vi "Configure Cells.vi"(8 "error in":errorcluster, 10 "dt":dbl, 11 "cCRDS in":refnum<class "cCRDS.lvclass">=refnum) -> (0 "error out":errorcluster, 3 "cCRDS out":refnum<class "cCRDS.lvclass">)   [LabVIEW 2015, in "cCRDS.lvclass"]
uses:
  cCRDS.lvclass
  Reusable/CRDS/Cell/CRDS Cell.lvclass
  Reusable/CRDS/Data/Cell/CRDS Cell Data.lvclass
  Reusable/CRDS/Data/Main/CRDS Data.lvclass
  Reusable/CRDS/Cell/Get Tau Method.ctl
  Data/cCRDS Data.lvclass
  Reusable/CRDS/Cell/CRDS Cell.lvclass/CRDS Cell.ctl
  Reusable/CRDS/Cell/Read Data.vi
  Reusable/CRDS/Cell/Write aVar Params.vi
  Reusable/CRDS/Cell/Write Data.vi
  Reusable/General/Atmospheric/Atmospheric Constants.vi
  Reusable/CRDS/Cell/Write CalType.vi
  Reusable/CRDS/Cell/Write errorCalOn.vi
  Reusable/CRDS/Cell/Write optTimeConst.vi
  Reusable/CRDS/Cell/Write dt.vi
  Reusable/CRDS/Cell/Write lambda.vi
  Reusable/CRDS/Data/Main/Write CellData.vi
  Reusable/CRDS/Main/Write Data.vi
  Reusable/CRDS/Main/Write Cells.vi
  Reusable/General/Atmospheric/Atmospheric Library.lvlib
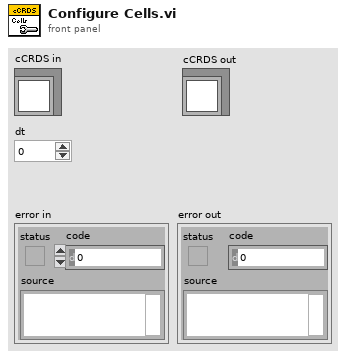
[diagram p1: front panel]
types:
  T1 = cluster{"tmeas":dbl, "tint":sgl[], "ttot":dbl, "Varaince On":bool}
  T2 = typedef "Get Tau Method.ctl" = enum8{"DFT-1", "DFT-5", "LRS"}
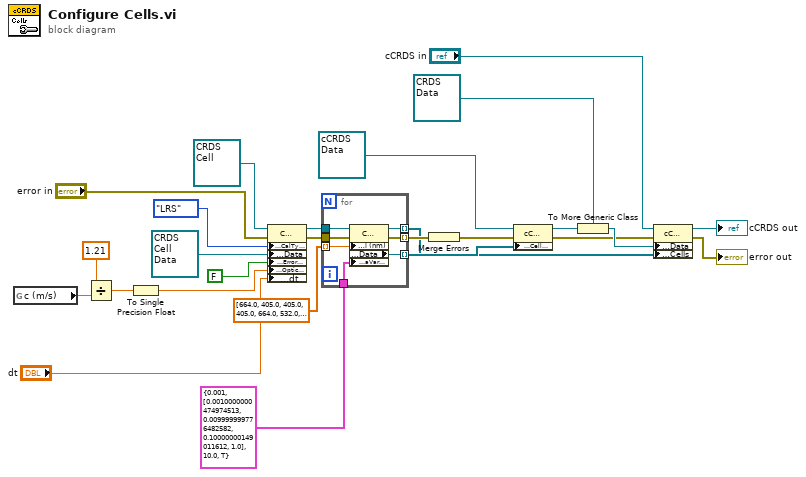
[diagram p0: block diagram]
diagram:
  n1 = global read "Atmospheric Constants.vi" "c (m/s)"() -> (w13:dbl)
  n2 = Divide(x=1.21, y=w13) -> (x/y=w14:dbl)
  n3 = To Single Precision Float(number=w14) -> (single precision float=w20:sgl)
  n4 = property class="CRDS Cell"(reference=refnum<class "CRDS Cell.lvclass"> refnum ("CRDS Cell"), error in="error in", "Data Access:CalType"=Get_Tau_Method."LRS" ("CalType"), "Data Access:Data"=refnum<class "CRDS Cell Data.lvclass"> refnum ("CRDS Cell"), "Data Access:Error Cal On?"=FALSE ("Error Cal On?"), "Data Access:Optical Time Constant"=w20, "Data Access:dt"="dt") -> (reference out=w21:refnum<class "CRDS Cell.lvclass">, error out=w22:errorcluster)
  n5 = for {
    tunnel: [w33] -> w9 mode=indexing
    tunnel: sgl[] [664.0, 405.0, 405.0, 405.0, 664.0, 532.0, 532.0, 532.0] -> [w31] mode=indexing
    tunnel: [w32] -> w24 mode=indexing
    tunnel: w21 -> [w30]
    tunnel: w22 -> [w29]
    tunnel: [w28] -> w26 mode=indexing
    tunnel: T1 {"tmeas"=0.001, "tint"=[0.001, 0.01, 0.1, 1.0], "ttot"=10.0, "Varaince On"=TRUE} ("aVar Params") -> [w27]
    n6 = property class="CRDS Cell"(reference=w30, error in=w29, "Data Access:l (nm)"=w31, "Data Access:aVar Params"=w27) -> (reference out=w33:refnum<class "CRDS Cell.lvclass">, error out=w32:errorcluster, "Data Access:Data"=w28:refnum<class "CRDS Cell Data.lvclass">)
  }
  n7 = Merge Errors(w24) -> (w8:errorcluster)
  n8 = property class="cCRDS Data"(reference=refnum<class "cCRDS Data.lvclass"> refnum ("cCRDS Data"), error in=w8, "Data Access:Cell Data"=w26) -> (reference out=w25:refnum<class "cCRDS Data.lvclass">, error out=w7:errorcluster)
  n9 = To More Generic Class(target class=refnum<class "CRDS Data.lvclass"> refnum ("Data"), reference=w25) -> (generic class reference=w10:refnum<class "CRDS Data.lvclass">)
  n10 = property class="cCRDS"(reference="cCRDS in", error in=w7, "Data Access:Data"=w10, "Data Access:Cells"=w9) -> (reference out=→"cCRDS out":refnum<class "cCRDS.lvclass">, error out=→"error out":errorcluster)
